vi "gfitsio-read-header.vi"(8 "error in (no error)":errorcluster, 11 "gfits refnum":T1) -> (0 "error out":errorcluster, 2 "header":string[](array[string]), 3 "dup gfits refnum":T1)   [LabVIEW 2023, in "gfitsio.lvlib"]
doc: "Return the entire header of the current HDU in an array of strings."
uses:
  gfitsio.lvlib
  gfitsio-refnum.ctl
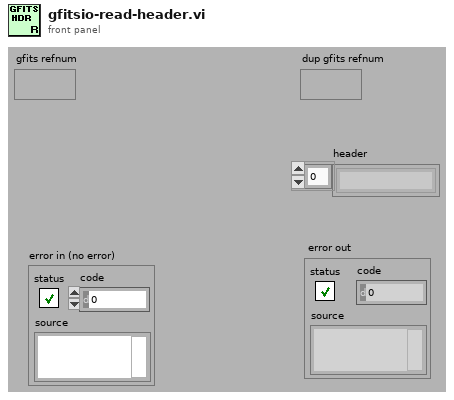
[diagram p1: front panel]
types:
  T1 = typedef "gfitsio.lvlib/gfitsio-refnum.ctl" = refnum<k1>
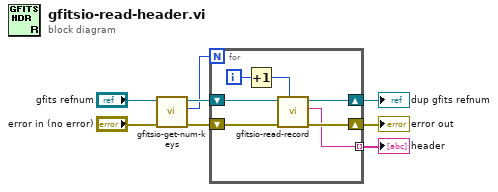
[diagram p0: block diagram]
diagram:
  n1 = call "gfitsio-get-num-keys.vi"("error in (no error)"="error in (no error)", "gfits refnum"="gfits refnum") -> ("error out"=w6:errorcluster, "number of keys"=w1:i32, "dup gfits refnum"=w5:T1)  [unwired: 7 out]
  n2 = for {
    N: w1 -> [_]
    shift-right: [w13] -> w4
    shift-left: w5 -> [w14]
    shift-right: [w12] -> w3
    shift-left: w6 -> [w15]
    tunnel: [w10] -> w2 mode=indexing
    i -> [w11]
    n3 = Increment(x=w11) -> (x+1=w9:i32)
    n4 = call "gfitsio-read-record.vi"("nrec"=w9, "error in (no error)"=w15, "gfits refnum"=w14) -> ("error out"=w12:errorcluster, "card"=w10:string, "dup gfits refnum"=w13:T1)  [unwired: 1 in, 5 out]
  }
  "error out" <- w3
  "dup gfits refnum" <- w4
  "header" <- w2
